vi "Add Message (BC to RT, RT to BC).vi"(4 "create timestamp channel":bool, 5 "message type":T1="BC to RT", 6 "parameters":T3(array[cluster]), 7 "number of words":u16=1, 8 "error in":errorcluster, 9 "remote terminal":T4, 10 "name":string, 11 "port in":T6 format="%.0x") -> (0 "error out":errorcluster, 3 "port out":T6 format="%.0x")   [LabVIEW 2020, in "Ballard MIL-STD-1553 Scripting.lvlib"]
uses:
  <vilib>/NI VeriStand/Custom Device API/Custom Device Item Ref.ctl
  Shared/Terminal Endpoint.ctl
  Shared/Address.ctl
  Shared/Parameter Definition.ctl
  Shared/Direction.ctl
  Ballard MIL-STD-1553 Scripting.lvlib
  <vilib>/NI VeriStand/Custom Device API/Custom Device API.lvlib
  Shared/Message Type.ctl
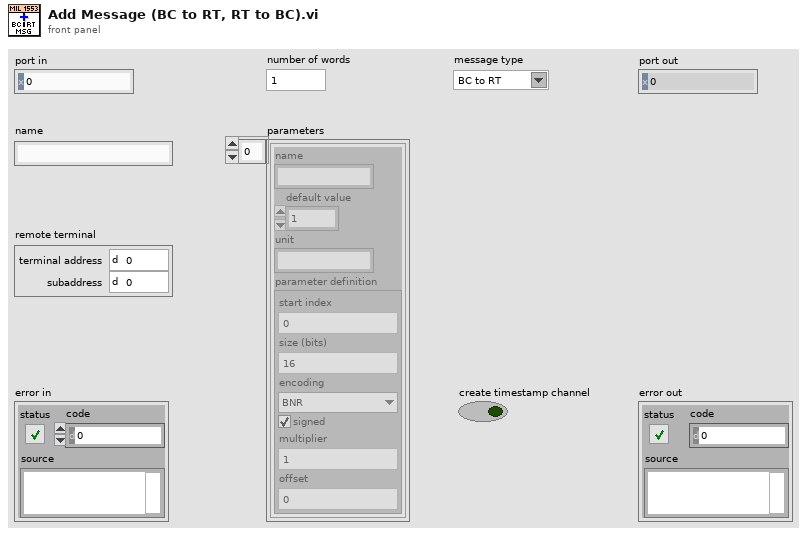
[diagram p1: front panel]
types:
  T1 = typedef "Message Type.ctl" = string
  T2 = typedef "Parameter Definition.ctl" = cluster{"start index":i32, "size (bits)":i32, "encoding":enum16{"BNR", "BCD", "Discrete"}, "signed":bool, "multiplier":dbl, "offset":dbl}
  T3 = cluster{"name":string, "default value":dbl, "unit":string, "parameter definition":T2}[]
  T4 = typedef "Terminal Endpoint.ctl" = cluster{"terminal address":T5, "subaddress":T5}
  T5 = typedef "Address.ctl" = u16
  T6 = typedef "Custom Device API.lvlib/Custom Device Item Ref.ctl" = u64
  T7 = typedef "Direction.ctl" = enum16{"Rx", "Tx"}
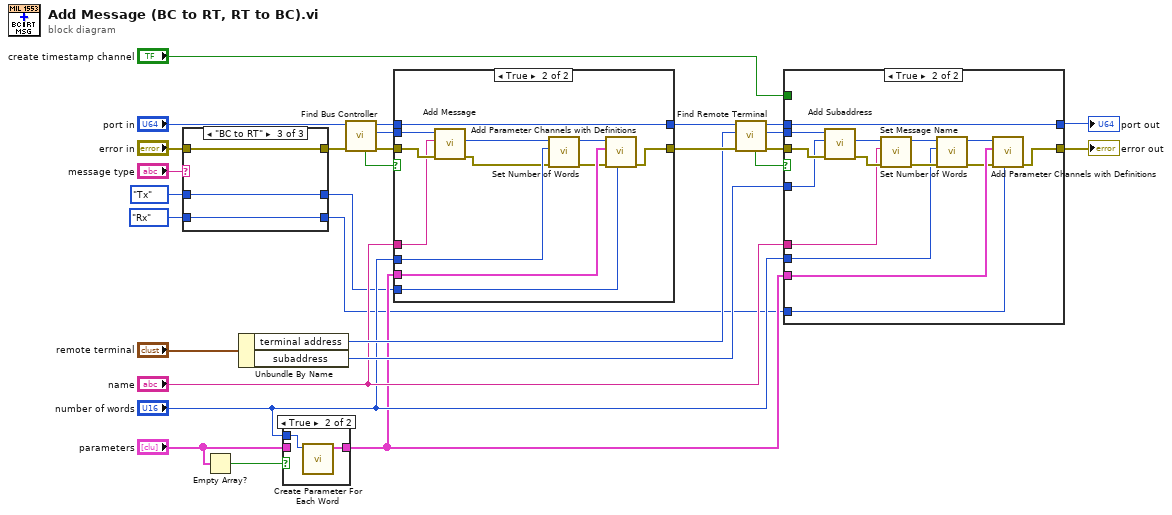
[diagram p0: block diagram]
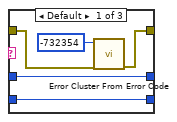
[diagram p2: hidden frame]
diagram:
  n1 = case shown="\"BC to RT\"" "message type" {
    tunnel: "error in" -> [w33 w37 w38]
    tunnel: Direction."Tx" -> [w31 w36 w40]
    tunnel: Direction."Rx" ("direction") -> [w30 w35 w39]
    tunnel: [w31 w35 w40] -> w3
    tunnel: [w30 w36 w39] -> w2
    tunnel: [w32 w37 w38] -> w1
    frame Default {
      n2 = call <vilib>:"Error Cluster From Error Code.vi"("error in (no error)"=w33, "error code (0)"=-732354) -> ("error out"=w32:errorcluster)  [unwired: 7 in]
    }
    frame "RT to BC" {
    }
    frame "BC to RT" {
    }
  }
  n3 = Empty Array?(array="parameters") -> (empty?=w12:bool)
  n4 = Unbundle By Name("remote terminal") -> ("terminal address"=w16:T5, "subaddress"=w14:T5)
  n5 = case shown="True" w12 {
    tunnel: "number of words" -> [_ w43]
    tunnel: "parameters" -> [w41 _]
    tunnel: [w41 w42] -> w9
    frame False {
    }
    frame True {
      n6 = call "Create Parameter For Each Word.vi"("number of words"=w43) -> ("parameters"=w42:T3)  [unwired: 9 in, 1 out]
    }
  }
  n7 = call "Find Bus Controller.vi"("error in"=w1, "port in"="port in") -> ("error out"=w25:errorcluster, "bus controller"=w26:T6, "port out"=w27:T6, "found?"=w28:bool)  [unwired: 6 in]
  n8 = case shown="True" w28 {
    tunnel: w27 -> [w45 w56]
    tunnel: w26 -> [_ w55]
    tunnel: w25 -> [w44 w57]
    tunnel: [w44 w53] -> w20
    tunnel: [w45 w56] -> w19
    tunnel: "number of words" -> [_ w54]
    tunnel: w9 -> [_ w52]
    tunnel: "name" -> [_ w47]
    tunnel: w3 -> [_ w46]
    frame False {
    }
    frame True {
      n9 = call "Add Message.vi"("error in"=w57, "message name"=w47, "bus controller in"=w55) -> ("error out"=w50:errorcluster, "message"=w51:T6)  [unwired: 6 in, 1 out]
      n10 = call "Set Number of Words.vi"("error in"=w50, "number of words"=w54, "message in"=w51) -> ("error out"=w48:errorcluster, "message out"=w49:T6)  [unwired: 7 in]
      n11 = call "Add Parameter Channels with Definitions.vi"("direction"=w46, "error in"=w48, "parameters"=w52, "message in"=w49) -> ("error out"=w53:errorcluster)  [unwired: 6 in, 1 out]
    }
  }
  n12 = call "Find Remote Terminal.vi"("error in"=w20, "terminal address"=w16, "port in"=w19) -> ("error out"=w24:errorcluster, "remote terminal"=w23:T6, "port out"=w22:T6, "found?"=w21:bool)  [unwired: 5 in]
  n13 = case shown="True" w21 {
    tunnel: w22 -> [w59 w73]
    tunnel: w23 -> [_ w72]
    tunnel: w24 -> [w58 w74]
    tunnel: [w58 w69] -> w17
    tunnel: [w59 w73] -> w18
    tunnel: w14 -> [_ w71]
    tunnel: "number of words" -> [_ w61]
    tunnel: w9 -> [_ w70]
    tunnel: "name" -> [_ w62]
    tunnel: "create timestamp channel" -> [_ _]
    tunnel: w2 -> [_ w60]
    frame False {
    }
    frame True {
      n14 = call "Add Subaddress.vi"("error in"=w74, "subaddress"=w71, "remote terminal in"=w72) -> ("error out"=w67:errorcluster, "subaddress ref"=w68:T6)  [unwired: 6 in, 1 out]
      n15 = call "Set Message Name.vi"("error in"=w67, "message name"=w62, "message in"=w68) -> ("error out"=w65:errorcluster, "message out"=w66:T6)  [unwired: 7 in]
      n16 = call "Set Number of Words.vi"("error in"=w65, "number of words"=w61, "message in"=w66) -> ("error out"=w63:errorcluster, "message out"=w64:T6)  [unwired: 7 in]
      n17 = call "Add Parameter Channels with Definitions.vi"("direction"=w60, "error in"=w63, "parameters"=w70, "message in"=w64) -> ("error out"=w69:errorcluster)  [unwired: 6 in, 1 out]
    }
  }
  "error out" <- w17
  "port out" <- w18
